vi "pulse generator for cal_training.vi"(0 "counter freq":u16=200, 1 "duty cylcle":dbl=0.5, 2 "clip length(sec)":sgl=1.0, 3 "error in":errorcluster, 4 "counter":tag="Dev1/ctr0") -> (7 "error out":errorcluster={"status"=TRUE, "code"=-200305, "source"="DAQmx Start Task.vi:7220004<append>\n<B>Property: </B>CO.Pulse.Freq\n<B>Corresponding Value: </B> 180.0\n\n<B>Property: </B>CO.Pulse.DutyCyc\n<B>Corresponding Value: </B> 500.0e-3\n\n<B>Property: </B>CO.Pulse.Freq.InitialDelay\n<B>Corresponding Value: </B> 0.0\n\n<B>Property: </B>CO.CtrTimebaseSrc\n<B>Corresponding Value: </B>/Dev1/MasterTimebase\n\n<B>Property: </B>SampQuant.SampPerChan\n<B>Corresponding Value: </B>180\n\n<B>Channel Name: </B>Dev1/ctr0\n\n<B>Task Name: </B>_unnamedTask<F>"})   [LabVIEW 2013]
doc: "I. Description:\nThis example demonstrates how to continuously output a waveform using an internal sample clock. The automatic regeneration of data has been disabled, so new data has to be provided throughout the duration of the continuous Analog Output operation. This allows the generation of any arbitrary frequency as this VI computes new data for each iteration of the loop, maintaining phase continuity of the signal.\n\nII. Instructions for Running:\n1. Select the Physical Channel to correspond to where your signal is output on the DAQ device.\n2. Enter the Minimum and Maximum Voltage range.\n3. Specify the desired Sample Clock Rate of the output Waveform. Higher sample clock rates will produce a smoother waveform.\n4. Manually specify the Analog Output buffer size, in number of samples. A larger buffer would help non-regenerative operations avoid errors due to occasional high CPU load. \nNote: \nThe Analog Output buffer has to be at least as big as the amount of data being written to the board per iteration. The recommended buffer size would be at least twice the amount of data being written to the board per iteration.\n5. Enter the Waveform Information. See the documentation of the Basic Function Generator SubVI for information on each parameter.\n\nIII. Block Diagram Steps:\n1. Create an Analog Output Voltage channel.\n2. Configure the task to prohibit the automatic regeneration of data.\n3. Call the DAQmx (Sample Clock) VI to set the sample clock rate. Additionally, set the sample mode to Continuous.\n4. Read the actual sample clock rate (eventually coerced depending on the hardware used). \n5. Compute the desired waveform, using the buffer size and the actual update rate. This VI keeps track of the phase of the waveform to ensure that the generated signal is continuous.\n6. Write the waveform to the output buffer. \n7a. Call the Start VI. This is only needed when the loop is executed for the first time.\n7b. Do nothing.\n8. Loop continuously until user presses the Stop button. Every iteration computes and writes a new waveform to the buffer.\n9. Call the Clear Task VI to clear the Task.\n10. Use the popup dialog box to display an error or warning if any.\n\nIV. I/O Connections Overview:\nMake sure your signal output terminal matches the Physical Channel I/O Control. For further connection information, refer to your hardware reference manual."
uses:
  <vilib>/DAQmx/create/channels.llb/DAQmx Create Channel (CO-Pulse Generation-Frequency).vi
  <vilib>/DAQmx/configure/timing.llb/DAQmx Timing (Implicit).vi
panel:
  out "AI refnum out":refnum<file>
  in  "stop":bool
  # "Counter Parameters"
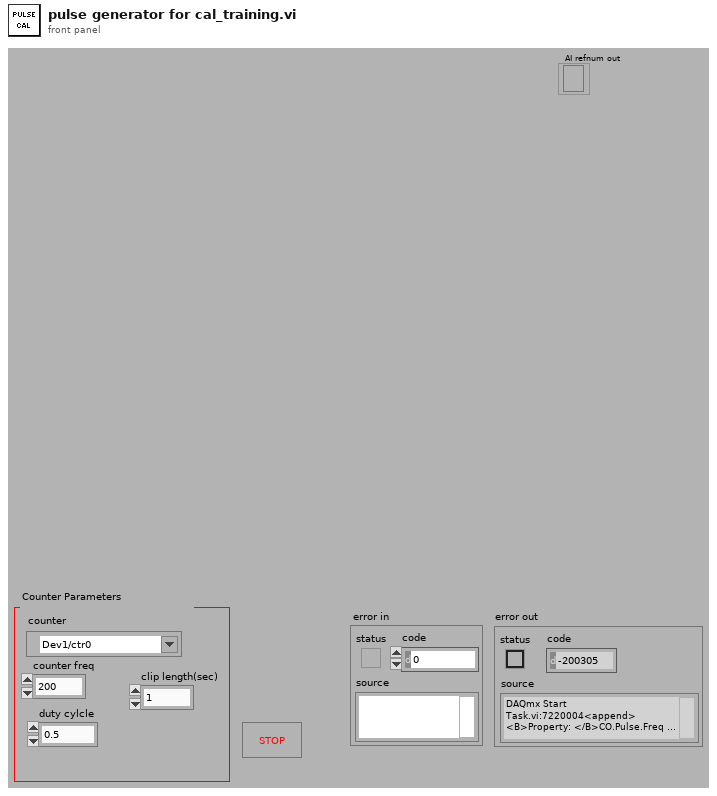
[diagram p1: front panel]
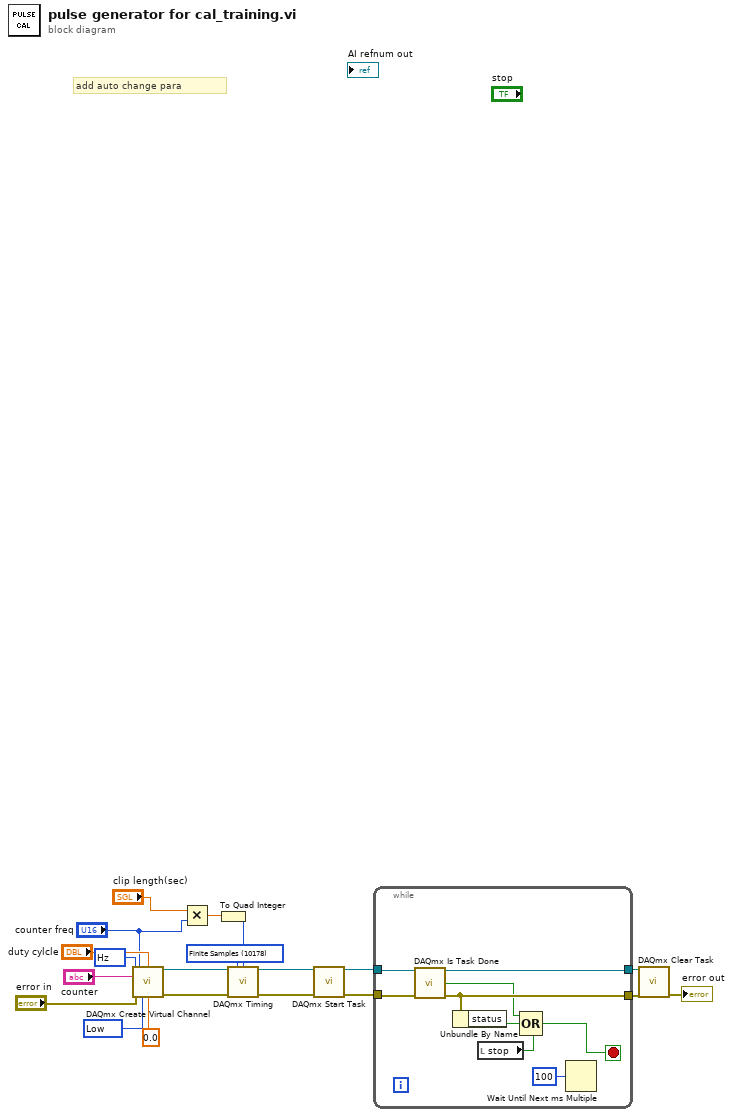
[diagram p0: block diagram]
diagram:
  w1 = 10373 items=["Hz"=10373] ("units")
  w15 = 10214 items=["High"=10192, "Low"=10214] ("idle state")
  w16 = 10178 items=["Finite Samples"=10178, "Continuous Samples"=10123, "Hardware Timed Single Point"=12522] ("sample mode")
  # "add auto change para"
  n1 = call-poly <vilib>:"DAQmx Create Virtual Channel.vi"("frequency"="counter freq", "duty cycle"="duty cylcle", "counter"="counter", "units"=w1, "error in"="error in", "idle state"=w15, "initial delay"=0.0) -> ("task out"=w17:refnum<k21>, "error out"=w18:errorcluster)  [unwired: 7 in]
  n2 = Multiply(x="clip length(sec)", y="counter freq") -> (x*y=w7:sgl)
  n3 = To Quad Integer(1:w7) -> (0:w6:i64)
  n4 = call-poly <vilib>:"DAQmx Timing.vi"("task/channels in"=w17, "sample mode"=w16, "samples per channel"=w6, "error in"=w18) -> ("task out"=w9:refnum<k21>, "error out"=w8:errorcluster)  [unwired: 10 in]
  n5 = call <vilib>:"DAQmx Start Task.vi"("task/channels in"=w9, "error in"=w8) -> ("task out"=w12:refnum<k21>, "error out"=w13:errorcluster)  [unwired: 12 in]
  n6 = while {
    tunnel: w13 -> [w28]
    tunnel: w12 -> [w29]
    tunnel: [w27] -> w11
    tunnel: [w26] -> w10
    stop <- w22 stop-if-true
    n7 = call <vilib>:"DAQmx Is Task Done.vi"("task/channels in"=w29, "error in"=w28) -> ("task out"=w27:refnum<k21>, "task done?"=w21:bool, "error out"=w26:errorcluster)  [unwired: 11 in]
    n8 = Unbundle By Name(w26) -> ("status"=w24:bool)
    n9 = local read "stop"() -> (w23:bool)
    n10 = Compound Arithmetic op=OR(w21, w24, w23) -> (w22:bool)
    n11 = Wait Until Next ms Multiple(millisecond multiple=u32 100) -> ()  [unwired: 1 out]
  }
  n12 = call <vilib>:"DAQmx Clear Task.vi"("task in"=w11, "error in"=w10) -> ("error out"=→"error out":errorcluster)  [unwired: 13 in]
